vi "Form GPS Sentence.vi"   [LabVIEW 2017, in "NMEA API.lvlib"]
doc: "Creates an NMEA sentence using the data you specify for a particular sentence type. You must manually select the polymorphic instance to use."
uses:
  <vilib>/robotics/Protocols/NMEA/NMEA API.lvlib
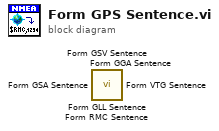
[diagram p0: block diagram]
diagram:
  n1 = call <vilib>:"Form GLL Sentence.vi"() -> ()  [unwired: 10 in, 2 out]
  n2 = call <vilib>:"Form GGA Sentence.vi"() -> ()  [unwired: 10 in, 2 out]
  n3 = call <vilib>:"Form GSA Sentence.vi"() -> ()  [unwired: 10 in, 2 out]
  n4 = call <vilib>:"Form VTG Sentence.vi"() -> ()  [unwired: 10 in, 2 out]
  n5 = call <vilib>:"Form RMC Sentence.vi"() -> ()  [unwired: 10 in, 2 out]
  n6 = call <vilib>:"Form GSV Sentence.vi"() -> ()  [unwired: 10 in, 2 out]
